vi "MicroPulse - system type and serial num decoder.vi"(9 "Extended Msg?":bool, 10 "RST Msg System Type in":u32 format="%.0x", 11 "RST Msg Serial # in":u64) -> (1 "System Type Enum":T1=enum."Micropulse 4", 2 "System Type String":string, 3 "Full Serial # out":u64)   [LabVIEW 2026, in "MicroPulse_Driver.lvlib"]
doc: "Decodes the system type from the values in the RST message. Adds a constant offset to the reported serial number based on system type.\n\nDecode of System type byte is as follows:\nBit 0 - 1: System Number MSB\nBit 2 - 3: For future use\nBit 4 - 7:\n0 = MicroPulse 5\n1 = MicroPulse LT1\n2 = MicroPulse LT2\n3 = LTPA\n4 = MPLT\n5 = MicroPulse 6\n\nPrevious models do not report a system type and will be assigned as a Micropulse 4.\n\nIf the incoming message is in the extended format (header: 0x2D46) then the \"Exended Msg?\" boolean input must be set to TRUE."
uses:
  MicroPulse_Driver.lvlib
  <instrlib>/MicroPulse/Public/Data/Datatypes/MP - instrument type.ctl
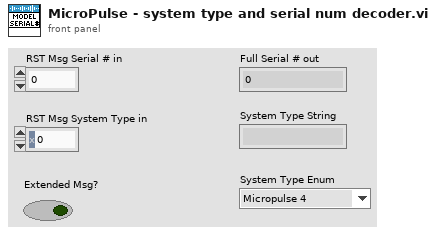
[diagram p1: front panel]
types:
  T1 = typedef "MicroPulse_Driver.lvlib/MP - instrument type.ctl" = enum16{"MicroPulse 5", "LT1", "LT2", "LTPA", "MPLT", "MicroPulse 6", "PipeScanner", "<MicroPulse>", "Micropulse 4", "Simulated Data"}
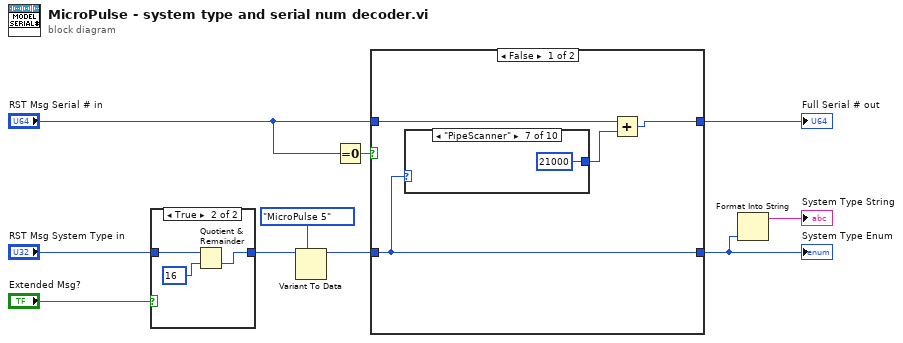
[diagram p0: block diagram]
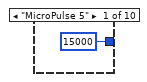
[diagram p3: hidden frame]
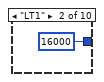
[diagram p4: hidden frame]
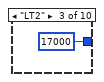
[diagram p5: hidden frame]
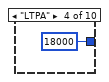
[diagram p6: hidden frame]
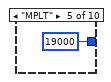
[diagram p7: hidden frame]
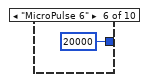
[diagram p8: hidden frame]
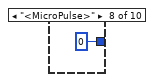
[diagram p9: hidden frame]
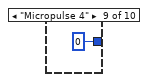
[diagram p10: hidden frame]
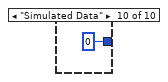
[diagram p11: hidden frame]
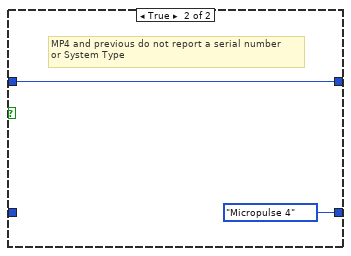
[diagram p12: hidden frame]
diagram:
  n1 = case shown="True" "Extended Msg?" {
    tunnel: "RST Msg System Type in" -> [w11 w14]
    tunnel: [w11 w13] -> w2
    frame False {
    }
    frame True {
      n2 = Quotient & Remainder(x=w14, y=u32 16 ("x")) -> (floor(x/y)=w13:u32)  [unwired: 1 out]
    }
  }
  n3 = Variant To Data(type=MP_-_instrument_type."MicroPulse 5" ("System Type"), Variant=w2) -> (data=w4:T1)  [unwired: 1 in, 1 out]
  n4 = Equal To 0?(x="RST Msg Serial # in") -> (x = 0?=w10:bool)
  n5 = case shown="False" w10 {
    tunnel: w4 -> [w15 _]
    tunnel: [w17 w30] -> w9
    tunnel: "RST Msg Serial # in" -> [w18 w30]
    tunnel: [w15 MP_-_instrument_type."Micropulse 4" ("System Type")] -> w6
    frame False {
      n6 = case shown="\"PipeScanner\"" w15 {
        tunnel: [u64 15000 ("RST Msg Serial # in") u64 16000 ("RST Msg Serial # in") u64 17000 ("RST Msg Serial # in") u64 18000 ("RST Msg Serial # in") u64 19000 ("RST Msg Serial # in") u64 20000 ("RST Msg Serial # in") u64 21000 ("RST Msg Serial # in") u64 0 ("RST Msg Serial # in") u64 0 ("RST Msg Serial # in") u64 0 ("RST Msg Serial # in")] -> w16
        frame "MicroPulse 5" {
        }
        frame "LT1" {
        }
        frame "LT2" {
        }
        frame "LTPA" {
        }
        frame "MPLT" {
        }
        frame "MicroPulse 6" {
        }
        frame "PipeScanner" {
        }
        frame "<MicroPulse>" {
        }
        frame "Micropulse 4" {
        }
        frame "Simulated Data" {
        }
      }
      n7 = Add(x=w18, y=w16) -> (x+y=w17:u64)
    }
    frame True {
      # "MP4 and previous do not report a serial number\nor System Type"
    }
  }
  "Full Serial # out" <- w9
  "System Type Enum" <- w6
  n8 = Format Into String(w6) -> (resulting string=→"System Type String":string)  [unwired: 3 in, 1 out]
